vi "ISEG_HVSystem.set Refresh Status.vi"(0 "i ref in":refnum<vi>, 2 "Refresh Status":dbl, 3 "Force":bool, 5 "error in (no error)":errorcluster) -> (14 "i ref out":refnum<vi>, 19 "error out":errorcluster)   [LabVIEW 2014, in "ISEG_HVSystem.lvlib"]
doc: "this vi set the default values for force_status and refresh rate."
uses:
  ISEG_HVSystem.lvlib
  CSCore/CSSystem/CoreLib/CoreLib.string 2 byte array.vi
  CSCore/CSSystem/CoreLib/CoreLib.short 2 byte array.vi
  CSCore/CSSystem/CoreLib/CoreLib.double 2 byte array.vi
  CSCore/CSSystem/CoreLib/CoreLib.lvlib
  CSCore/BaseProcess/BaseProcess.lvlib
  CSlibraries-extern/DimLVEvent/LVDimInterface/LVDimInterface.lvlib
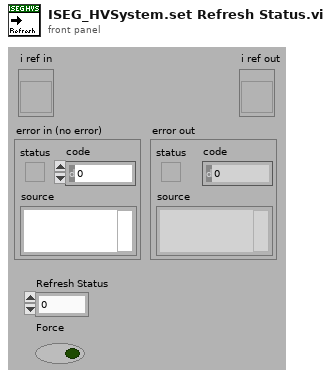
[diagram p1: front panel]
types:
  T1 = typedef "BaseProcess.lvlib/BaseProcess.i attribute.ctl" = cluster{"EventStatus":string, "EventError":i32, "PresetEvtWatchD":i32, "PresetPdcWatchD":i32, "EventTimeout":i32, "PeriodicInterval":i32, "Interface":string[], "Address":string[], "Special":string[], "PeriodicError":i32, "PeriodicStatus":string, "SuperProc":string, "Descriptors":T2[], "CaseRef":refnum<vi>, "PdcRef":refnum<vi>, "Thread Ref":refnum<vi>, "eventErrorID":i32, "eventStatusID":i32, "periodicErrorID":i32, "periodicStatusID":i32, "pdcCtrID":i32}
  T2 = typedef "BaseProcess.lvlib/BaseProcess.descriptor definition.ctl" = cluster{"selector":string, "descriptor":T3}
  T3 = typedef "BaseProcess.lvlib/BaseProcess.descriptor string definition.ctl" = string
  T4 = typedef "CoreDefs.rawDataType.ctl" = i8[]
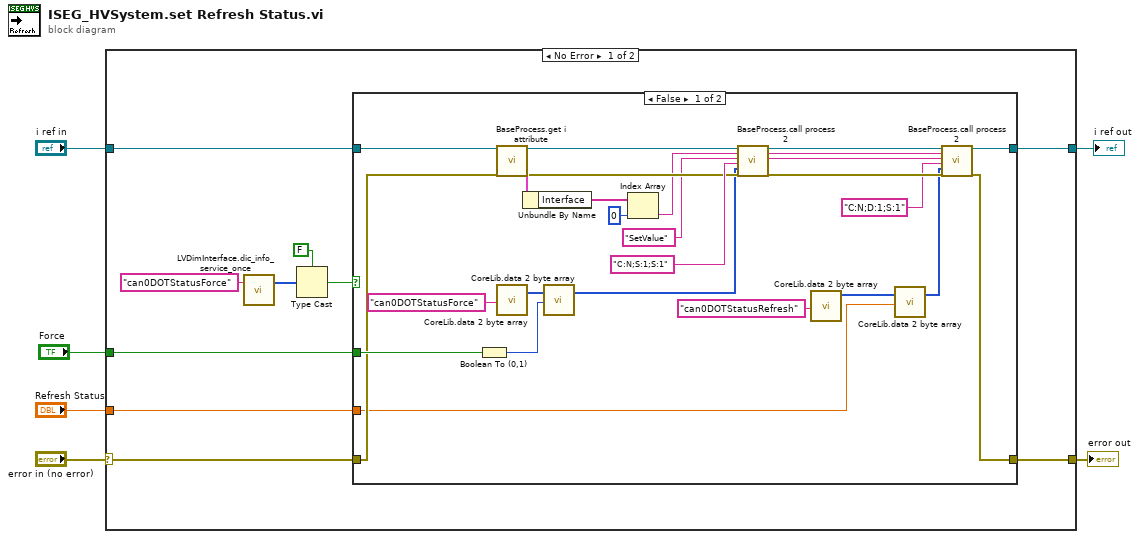
[diagram p0: block diagram]
diagram:
  n1 = case shown="No Error" "error in (no error)" {
    selector: "error in (no error)" -> [w7 w43]
    tunnel: "i ref in" -> [w16 w44]
    tunnel: "Refresh Status" -> [w15 _]
    tunnel: "Force" -> [w12 _]
    tunnel: [w14 w44] -> w2
    tunnel: [w13 w43] -> w1
    frame No Error {
      n2 = call "LVDimInterface.dic_info_service_once.vi"("serviceName"="can0DOTStatusForce") -> ("data"=w9:i8[])  [unwired: 15 in, 3 out]
      n3 = Type Cast(type=FALSE, x=w9) -> (*(type *) &x=w8:bool)
      n4 = case shown="False" w8 {
        tunnel: w16 -> [w40 w42]
        tunnel: w15 -> [w18 _]
        tunnel: [w32 w42] -> w14
        tunnel: [w30 w41] -> w13
        tunnel: w12 -> [w24 _]
        tunnel: w7 -> [w23 w41]
        frame False {
          w28 = "SetValue" ("Selector")
          n5 = Boolean To (0,1)(Boolean=w24) -> (0, 1=w21:i16)
          n6 = call "BaseProcess.get i attribute.vi"("i ref in"=w40, "error in (no error)"=w23) -> ("i ref out"=w35:refnum<vi>, "i attribute"=w37:T1, "error out"=w34:errorcluster)  [unwired: 15 in]
          n7 = call-poly "CoreLib.data 2 byte array.vi"("string"="can0DOTStatusForce") -> ("byteArray out"=w22:T4)  [unwired: 18 in]
          n8 = Unbundle By Name(w37) -> ("Interface"=w39:string[])
          n9 = call-poly "CoreLib.data 2 byte array.vi"("byteArray"=w22, "i16"=w21) -> ("byteArray out"=w20:T4)  [unwired: 17 in]
          n10 = Index Array(array=w39, index=0) -> (element=w29:string)
          n11 = call "BaseProcess.call process 2.vi"("i ref in"=w35, "Object"=w29, "Selector"=w28, "Data Descriptor"="C:N;S:1;S:1", "Data"=w20, "error in (no error)"=w34) -> ("i ref out"=w33:refnum<vi>, "error out"=w31:errorcluster)  [unwired: 12 in]
          n12 = call-poly "CoreLib.data 2 byte array.vi"("string"="can0DOTStatusRefresh") -> ("byteArray out"=w19:T4)  [unwired: 18 in]
          n13 = call-poly "CoreLib.data 2 byte array.vi"("byteArray"=w19, "f64"=w18) -> ("byteArray out"=w17:T4)  [unwired: 17 in]
          n14 = call "BaseProcess.call process 2.vi"("i ref in"=w33, "Object"=w29, "Selector"=w28, "Data Descriptor"="C:N;D:1;S:1", "Data"=w17, "error in (no error)"=w31) -> ("i ref out"=w32:refnum<vi>, "error out"=w30:errorcluster)  [unwired: 12 in]
        }
        frame True {
        }
      }
    }
    frame Error {
    }
  }
  "error out" <- w1
  "i ref out" <- w2
